vi "RunMeSomeTests.vi"(8 "error in (no error)":errorcluster, 11 "Caraya-TestableClass in":refnum<class "Caraya-TestableClass.lvclass">) -> (0 "error out":errorcluster, 3 "Caraya-TestableClass out":refnum<class "Caraya-TestableClass.lvclass">)   [LabVIEW 2020, in "Caraya-TestableClass.lvclass"]
uses:
  Caraya-TestableClass.lvclass
  Caraya-TestableClass.lvclass/Caraya-TestableClass.ctl
  classes/Test/Test.lvclass
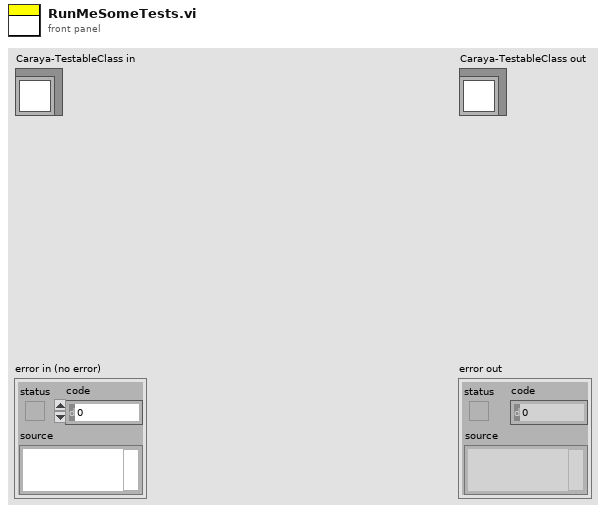
[diagram p1: front panel]
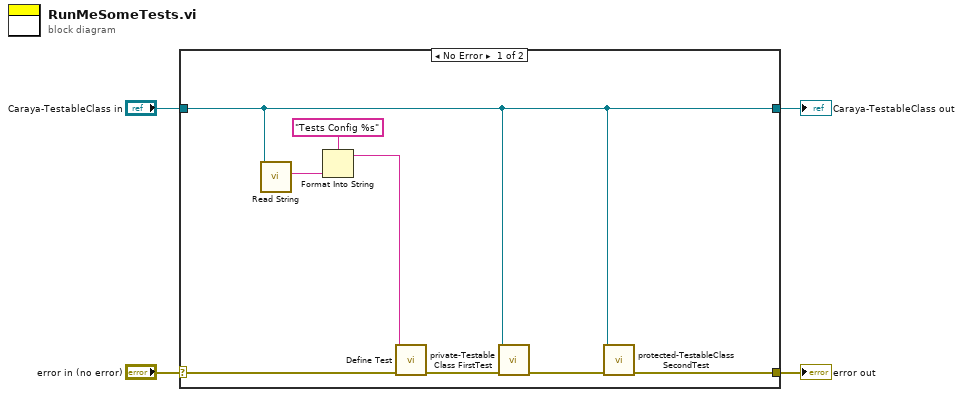
[diagram p0: block diagram]
diagram:
  n1 = case shown="No Error" "error in (no error)" {
    selector: "error in (no error)" -> [w10 w14]
    tunnel: [w11 w14] -> w3
    tunnel: [w5 w13] -> w1
    tunnel: "Caraya-TestableClass in" -> [w5 w13]
    frame No Error {
      n2 = call "Read String.vi"("Caraya-TestableClass in"=w5) -> ("String"=w8:string)  [unwired: 9 in, 1 out]
      n3 = Format Into String(format string="Tests Config %s", w8) -> (resulting string=w6:string)  [unwired: 2 in, 1 out]
      n4 = call "Define Test.vi"("error in (no error)"=w10, "Label (VI Title)"=w6) -> ("error out"=w9:errorcluster)  [unwired: 8 in, 1 out]
      n5 = call "private-TestableClass FirstTest.vi"("error in (no error)"=w9, "Caraya-TestableClass in"=w5) -> ("error out"=w12:errorcluster)  [unwired: 9 in]
      n6 = call "protected-TestableClass SecondTest.vi"("error in (no error)"=w12, "Caraya-TestableClass in"=w5) -> ("error out"=w11:errorcluster)  [unwired: 9 in]
    }
    frame Error {
    }
  }
  "error out" <- w3
  "Caraya-TestableClass out" <- w1
